vi "VerifyFile.vi"(11 "File to save":path) -> (0 "error out":errorcluster, 3 "selected path":path)   [LabVIEW 2016]
doc: "verify that the given path is a valid path, if it isn't a valid path, asks user for a path. if user cancelled, outputs an error"
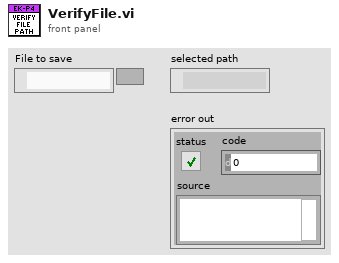
[diagram p1: front panel]
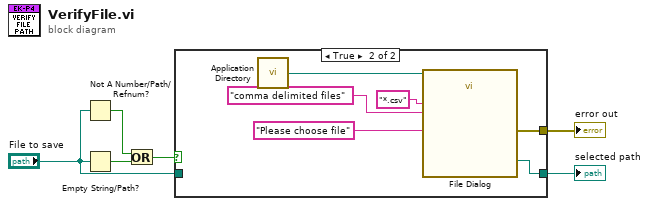
[diagram p0: block diagram]
diagram:
  n1 = Not A Number/Path/Refnum?(number/path/refnum="File to save") -> (NaN/Path/Refnum?=w3:bool)
  n2 = Empty String/Path?(string/path="File to save") -> (empty?=w2:bool)
  n3 = Or(x=w3, y=w2) -> (x .or. y?=w1:bool)
  n4 = case shown="True" w1 {
    tunnel: [w7 w13] -> w6
    tunnel: "File to save" -> [w7 _]
    tunnel: [_ w9] -> w5
    frame False {
    }
    frame True {
      n5 = call <vilib>:"Application Directory.vi"() -> ("Application Directory"=w8:path)
      n6 = call "File Dialog"("start path"=w8, "prompt"="Please choose file", "pattern (all files)"="*.csv", "pattern label"="comma delimited files") -> ("selected path"=w13:path, "error out"=w9:errorcluster)  [unwired: 8 in, 2 out]
    }
  }
  "selected path" <- w6
  "error out" <- w5
